vi "제목없음 1.vi"() -> ()   [LabVIEW 2018]
panel:
  out "부정 차트 4":dbl(graph)
  out "복합 차트 3":dbl(graph)
  out "중립 차트 2":dbl(graph)
  out "긍정 차트":dbl(graph)
  out "반환값":string[](array[string])
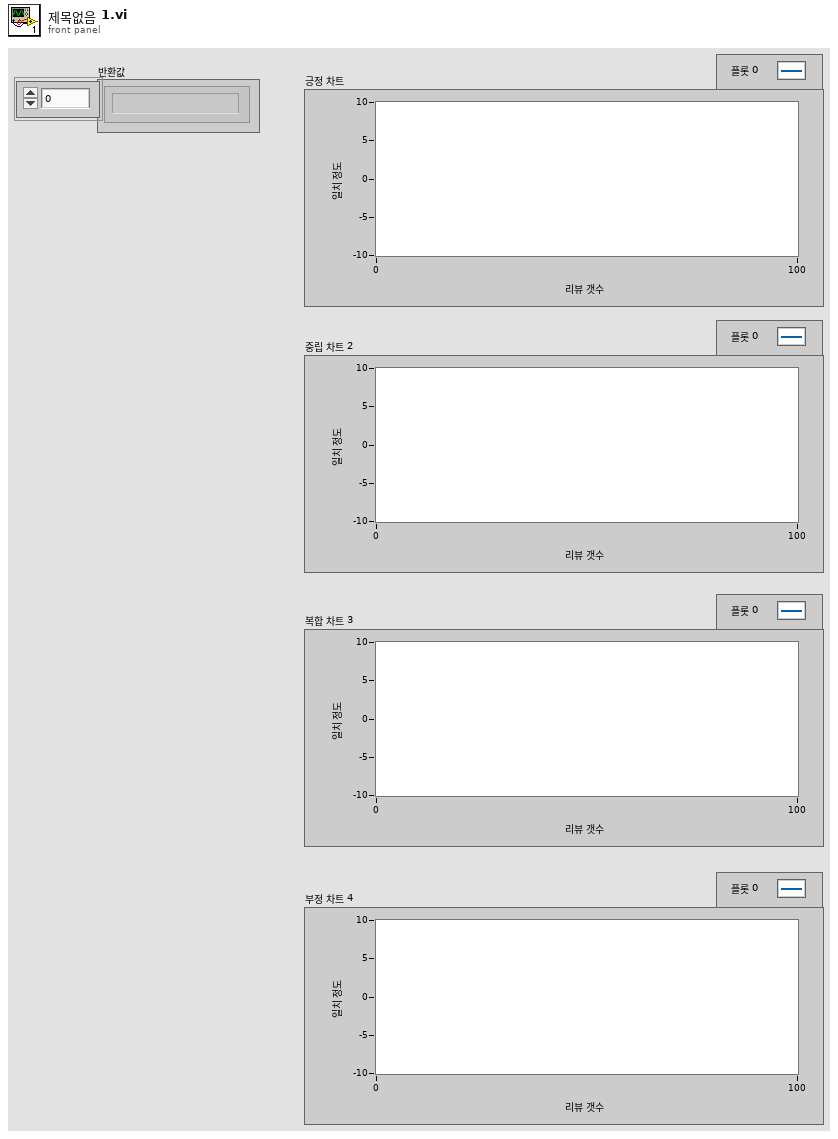
[diagram p1: front panel]
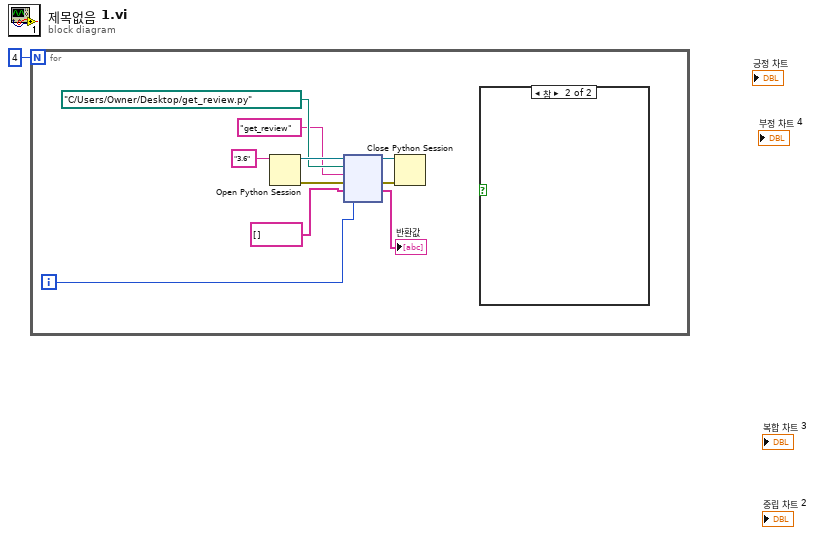
[diagram p0: block diagram]
diagram:
  n1 = for {
    N: 4 -> [_]
    i -> [w2]
    n2 = Open Python Session(python version="3.6" ("Python 버전")) -> (session out=w9:refnum<k35>, error out=w10:errorcluster)  [unwired: 2 in]
    n3 = node(w9, path "C:/Users/Owner/Desktop/get_review.py" ("모듈 경로"), "get_review" ("함수 이름"), w10, string[] [], w2) -> (w8:refnum<k35>, w7:errorcluster, →"반환값":string[])  [unwired: 1 in, 2 out]
    n4 = Close Python Session(session in=w8, error in=w7) -> ()  [unwired: 1 out]
    n5 = case shown="참" {
      selector: _ -> [_ _]
      frame False {
      }
      frame True {
      }
    }
  }
